vi "Recursive Folder List.vi"(4 "Folders to Exclude":string[](array[string]), 6 "pattern":string, 8 "error in (no error)":errorcluster, 9 "Continue Recursing on Error? (F)":bool, 11 "Folder Path":path) -> (0 "error out":errorcluster, 1 "Number of Files":i32, 2 "All Files in Dir":path[](array[path]), 3 "dup Folder Path":path, 5 "All Folders":path[](array[path]))   [LabVIEW 2017]
doc: "Lists the contents of a folder or LLB."
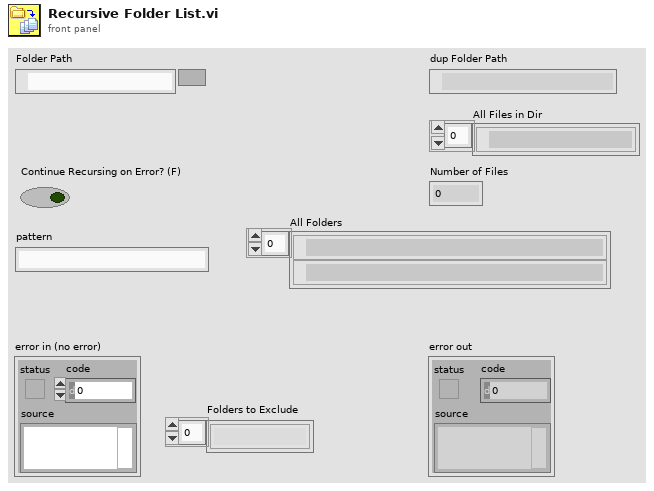
[diagram p1: front panel]
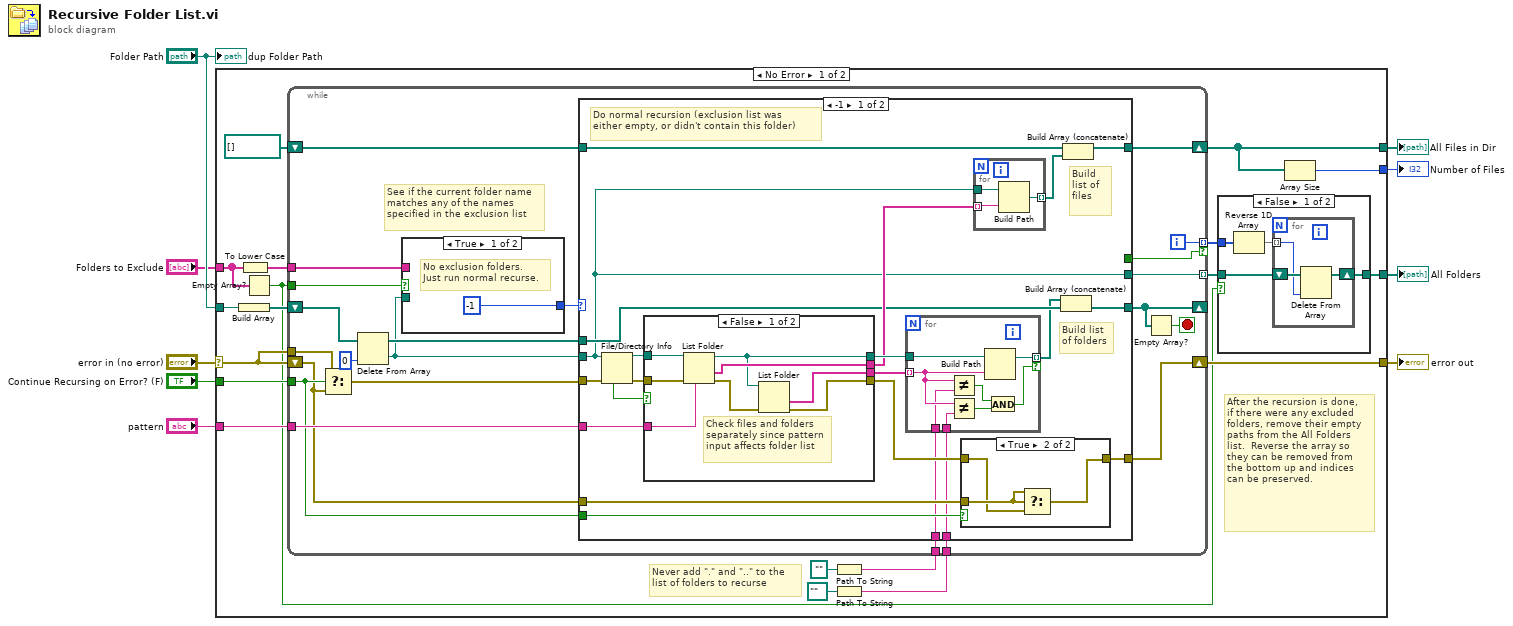
[diagram p0: block diagram]
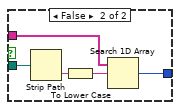
[diagram p2: hidden frame]
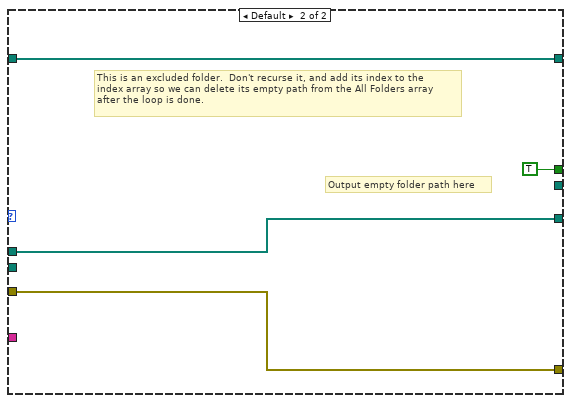
[diagram p5: hidden frame]
diagram:
  n1 = case shown="No Error" "error in (no error)" {
    selector: "error in (no error)" -> [w20 w115]
    tunnel: "Folder Path" -> [w28 _]
    tunnel: [w23 _] -> w9
    tunnel: [w22 _] -> w8
    tunnel: [w24 w115] -> w7
    tunnel: [w17 _] -> w5
    tunnel: "pattern" -> [w25 _]
    tunnel: "Continue Recursing on Error? (F)" -> [w21 _]
    tunnel: "Folders to Exclude" -> [w15 _]
    frame No Error {
      # "Never add \".\" and \"..\" to the list of folders to recurse"
      # "After the recursion is done,\nif there were any excluded\nfolders, remove their empty\npaths from the All Folders\nlist.  Reverse the array so\nthey can be removed from\nthe bottom up and indices\ncan be preserved."
      n2 = Build Array(w28) -> (w27:path[])
      n3 = To Lower Case(string=w15) -> (all lower case string=w19:string[])
      n4 = Empty Array?(array=w15) -> (empty?=w14:bool)
      n5 = Path To String(path=path "") -> (string=w11:string)
      n6 = Path To String(path=path "..") -> (string=w10:string)
      n7 = while {
        shift-left: path[] [] ("Array Constant") -> [w48]
        shift-right: [w50] -> w23
        shift-left: w27 -> [w49]
        shift-right: [w46] -> _
        shift-right: [w40] -> w24
        shift-left: w20 -> [w39]
        tunnel: [w37] -> w18 mode=indexing
        tunnel: w25 -> [w47]
        tunnel: w21 -> [w41]
        tunnel: w20 -> [w42]
        tunnel: w19 -> [w35]
        tunnel: w14 -> [w36]
        tunnel: [w32] -> w16 mode=indexing if=w31
        tunnel: w11 -> [w30]
        tunnel: w10 -> [w29]
        i -> [w32]
        stop <- w45 stop-if-true
        # "See if the current folder name\nmatches any of the names\nspecified in the exclusion list"
        n8 = Select(t=w42, s=w41, f=w39) -> (s? t:f=w43:errorcluster)
        n9 = Delete From Array(array=w49, index=0) -> (deleted portion=w34:path, array with subset deleted=w38:path[])  [unwired: 1 in]
        n10 = case shown="True" w36 {
          tunnel: w35 -> [_ w53]
          tunnel: w34 -> [_ w56]
          tunnel: [-1 ("index of element") w52] -> w33
          frame True {
            # "No exclusion folders.\nJust run normal recurse."
          }
          frame False {
            n11 = Strip Path(path=w56) -> (name=w55:string)  [unwired: 1 out]
            n12 = To Lower Case(string=w55) -> (all lower case string=w54:string)
            n13 = Search 1D Array(1D array=w53, element=w54) -> (index of element=w52:i32)  [unwired: 1 out]
          }
        }
        n14 = case shown="-1" w33 {
          tunnel: [w77 w106] -> w50
          tunnel: w48 -> [w76 w106]
          tunnel: w47 -> [w74 _]
          tunnel: [w72 w105] -> w46
          tunnel: w34 -> [w61 _]
          tunnel: w43 -> [w68 w104]
          tunnel: w41 -> [w66 _]
          tunnel: [w65 w104] -> w40
          tunnel: w39 -> [w64 _]
          tunnel: w38 -> [w62 w105]
          tunnel: [w61 _] -> w37
          tunnel: [_ TRUE] -> w31
          tunnel: w30 -> [w58 _]
          tunnel: w29 -> [w57 _]
          frame -1 {
            # "Build list of files"
            # "Build list\nof folders"
            # "Do normal recursion (exclusion list was\neither empty, or didn't contain this folder)"
            n15 = File/Directory Info(path=w61, error in=w68) -> (path out=w70:path, error out=w71:errorcluster, shortcut=w69:bool)  [unwired: 4 out]
            n16 = case shown="False" w69 {
              tunnel: [w93 _] -> w63
              tunnel: [w92 w95] -> w75
              tunnel: [w91 w94] -> w67
              tunnel: w74 -> [w90 _]
              tunnel: [w86 _] -> w73
              tunnel: w71 -> [w89 w94]
              tunnel: w70 -> [w88 w95]
              frame False {
                # "Check files and folders\nseparately since pattern\ninput affects folder list"
                n17 = List Folder(path=w88, pattern=w90, error in=w89) -> (path out=w92:path, folder names=w93:string[], error out=w87:errorcluster)  [unwired: 2 out]
                n18 = List Folder(path=w92, error in=w87) -> (folder names=w86:string[], error out=w91:errorcluster)  [unwired: 4 out]
              }
              frame True {
                # "Do not attempt to recurse the contents of folder shortcuts"
              }
            }
            n19 = for {
              tunnel: w75 -> [w85]
              tunnel: [w84] -> w60 mode=indexing if=w83
              tunnel: w73 -> [w82] mode=indexing
              tunnel: w58 -> [w81]
              tunnel: w57 -> [w80]
              n20 = Not Equal?(x=w82, y=w81) -> (x != y?=w78:bool)
              n21 = Not Equal?(x=w82, y=w80) -> (x != y?=w79:bool)
              n22 = Build Path(base path=w85, name or relative path=w82) -> (appended path=w84:path)
              n23 = And(x=w78, y=w79) -> (x .and. y?=w83:bool)
            }
            n24 = case shown="True" w66 {
              tunnel: w67 -> [w99 w101]
              tunnel: [w99 w100] -> w65
              tunnel: w64 -> [_ w102]
              frame False {
              }
              frame True {
                n25 = Select(t=w102, s=w102, f=w101) -> (s? t:f=w100:errorcluster)
              }
            }
            n26 = for {
              tunnel: w63 -> [w97] mode=indexing
              tunnel: w61 -> [w98]
              tunnel: [w96] -> w59 mode=indexing
              n27 = Build Path(base path=w98, name or relative path=w97) -> (appended path=w96:path)
            }
            n28 = Build Array (concatenate)(w60, w62) -> (w72:path[])
            n29 = Build Array (concatenate)(w76, w59) -> (w77:path[])
          }
          frame Default {
            # "Output empty folder path here"
            # "This is an excluded folder.  Don't recurse it, and add its index to the\nindex array so we can delete its empty path from the All Folders array\nafter the loop is done."
          }
        }
        n30 = Empty Array?(array=w46) -> (empty?=w45:bool)
      }
      n31 = case shown="False" w14 {
        tunnel: w18 -> [w109 w114]
        tunnel: [w108 w114] -> w17
        tunnel: w16 -> [w110 _]
        frame False {
          n32 = Reverse 1D Array(array=w110) -> (reversed array=w107:i32[])
          n33 = for {
            shift-right: [w112] -> w108
            shift-left: w109 -> [w113]
            tunnel: w107 -> [w111] mode=indexing
            n34 = Delete From Array(array=w113, index=w111) -> (array with subset deleted=w112:path[])  [unwired: 1 in, 1 out]
          }
        }
        frame True {
          # "No excluded folders.\nDon't run the code that\ndeletes excluded folder\nindices."
        }
      }
      n35 = Array Size(array=w23) -> (size(s)=w22:i32)
    }
    frame Error {
    }
  }
  "All Files in Dir" <- w9
  "Number of Files" <- w8
  "error out" <- w7
  "All Folders" <- w5
  "dup Folder Path" <- "Folder Path"
